vi "Flat.vi"(11 "File Path":path=path "C:/Users/STED/Desktop/Cambridge STED Control Software/Host VIs/SLM/Flatness Correction LSH0700935/CAL_LSH0700935_770nm.bmp") -> (2 "Flatness":dbl[][](array[numeric]))   [LabVIEW 2018]
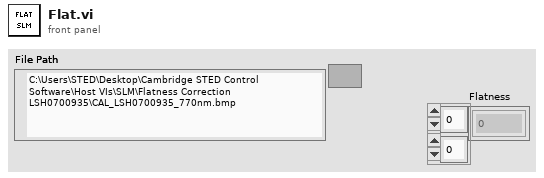
[diagram p1: front panel]
types:
  T1 = typedef "IMAQ Image.ctl" = refnum<image>
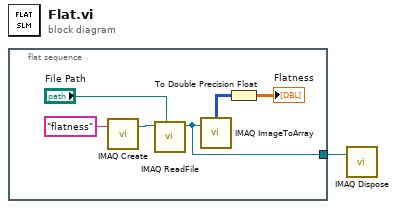
[diagram p0: block diagram]
diagram:
  n1 = flat-sequence {
    tunnel: [w2] -> w1
    frame #0 {
      n2 = call "IMAQ Create"("Image Name"="flatness") -> ("New Image"=w7:T1)  [unwired: 3 in, 2 out]
      n3 = call "IMAQ ReadFile"("File Path"="File Path", "Image"=w7) -> ("Image Out"=w2:T1)  [unwired: 3 in, 6 out]
      n4 = call "IMAQ ImageToArray"("Image"=w2) -> ("Image Pixels (U8)"=w5:u8[][])  [unwired: 2 in, 5 out]
      n5 = To Double Precision Float(number=w5) -> (double precision float=→"Flatness":dbl[][])
    }
  }
  n6 = call "IMAQ Dispose"("Image"=w1) -> ()  [unwired: 5 in, 1 out]
